vi "Agilent B2900 Series Output User Defined Waveform.vi"() -> ()   [LabVIEW 2023]
doc: "This example shows how to use the instrument's output user defined waveform.\n\n<B>Note:</B>\nThis example is only supported by Agilent models B2961A, B2962A, B2961B and B2962B."
uses:
  Agilent B2900 Series.lvlib
panel:
  in  "Enable Trigger Output (T: Enable)":bool=TRUE
  in  "Trigger Output Port (0: External1)":i32(ring) items=["External1", "External2", "External3", "External4", "External5", "External6", "External7", "External8", "External9", "External10", "External11", "External12", "External13", "External14", "Internal1", "Internal2"]
  in  "Step Time (1E-5 seconds)":dbl=1e-05
  in  "List Trigger Output":bool[](array[boolean])=[TRUE, TRUE, FALSE, TRUE]
  in  "List Output Data":dbl[](array[numeric])=[0.1, 0.2, 0.3, 0.1]
  out "OCP Tripped?":bool
  in  "Enable Output Protection(T: Enable)":bool=TRUE
  in  "Compliance Current (0.0001 A)":dbl=0.0001 format="%_3g"
  in  "Output Channel (0: Channel 1)":i32(ring) items=["Channel 1", "Channel 2"]
  in  "VISA resource name":refnum<visa-resource-name>
  # "(c) 2011-2021 National Instruments.  ALL RIGHTS RESERVED."
  # "Compliance Protection"
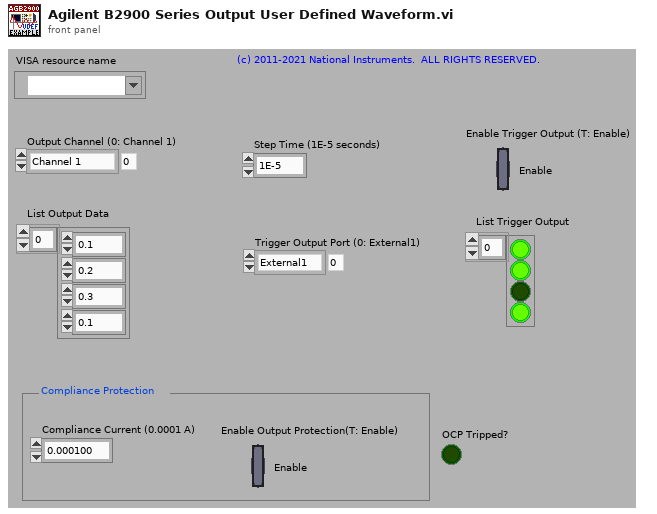
[diagram p1: front panel]
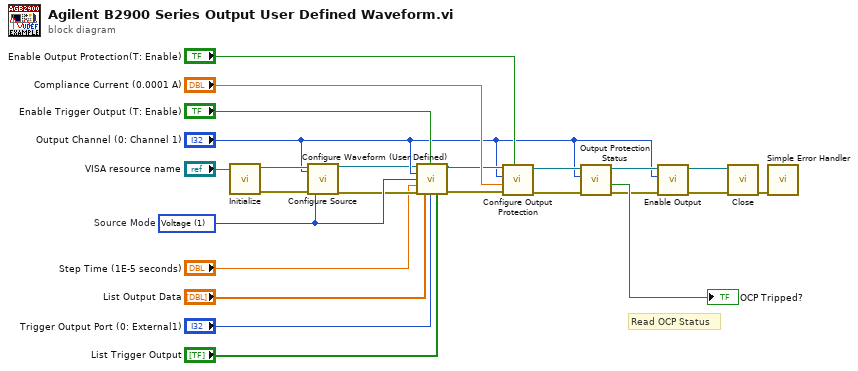
[diagram p0: block diagram]
diagram:
  w7 = 1 items=["Current", "Voltage"]  # Source Mode
  # "Read OCP Status"
  n1 = call "Initialize.vi"("VISA resource name"="VISA resource name") -> ("error out"=w18:errorcluster, "VISA resource name out"=w19:refnum<visa-resource-name>)  [unwired: 9 in]
  n2 = call "Configure Source.vi"("VISA resource name"=w19, "Channel (0: Channel 1)"="Output Channel (0: Channel 1)", "error in (no error)"=w18, "Source Mode (1: Voltage)"=w7) -> ("VISA resource name out"=w6:refnum<visa-resource-name>, "error out"=w5:errorcluster)  [unwired: 14 in]
  n3 = call "Configure Waveform (User Defined).vi"("VISA resource name"=w6, "Enable Trigger Output (T: Enable)"="Enable Trigger Output (T: Enable)", "Output Channel (0: Channel 1)"="Output Channel (0: Channel 1)", "Source Mode (1: Voltage)"=w7, "Step Time (1E-5 seconds)"="Step Time (1E-5 seconds)", "error in (no error)"=w5, "List Of Output Data"="List Output Data", "Trigger Output Port (0: External1)"="Trigger Output Port (0: External1)", "List Of Trigger Output"="List Trigger Output") -> ("VISA resource name out"=w11:refnum<visa-resource-name>, "error out"=w10:errorcluster)  [unwired: 5 in]
  n4 = call "Configure Output Protection.vi"("Enable Output Protection (T: Enable)"="Enable Output Protection(T: Enable)", "error in (no error)"=w10, "Compliance Current (0.0001 A)"="Compliance Current (0.0001 A)", "Channel (0: Channel 1)"="Output Channel (0: Channel 1)", "VISA resource name"=w11) -> ("error out"=w16:errorcluster, "VISA resource name out"=w17:refnum<visa-resource-name>)  [unwired: 5 in]
  n5 = call "Output Protection Status.vi"("error in (no error)"=w16, "Channel (0: Channel 1)"="Output Channel (0: Channel 1)", "VISA resource name"=w17) -> ("error out"=w14:errorcluster, "OCP Tripped?"=→"OCP Tripped?":bool, "VISA resource name out"=w15:refnum<visa-resource-name>)  [unwired: 5 in, 1 out]
  n6 = call "Enable Output.vi"("error in (no error)"=w14, "Channel (0: Channel 1)"="Output Channel (0: Channel 1)", "VISA resource name"=w15) -> ("error out"=w12:errorcluster, "VISA resource name out"=w13:refnum<visa-resource-name>)  [unwired: 6 in, 1 out]
  n7 = call "Close.vi"("error in (no error)"=w12, "VISA resource name"=w13) -> ("error out"=w23:errorcluster)  [unwired: 9 in]
  n8 = call <vilib>:"Simple Error Handler.vi"("error in (no error)"=w23) -> ()  [unwired: 4 in, 5 out]
